vi "Sub_post_processing.vi"(0 "Experiment":T1, 1 "file name":i32, 2 "Save Acceleration Data":bool) -> (7 "Frequency":waveform(dbl)[](array[waveform]), 8 "Position":waveform(dbl)[](array[waveform]), 9 "average cycle time (ms)":dbl=4.283940110367686 format="%0.2f")   [LabVIEW 2021]
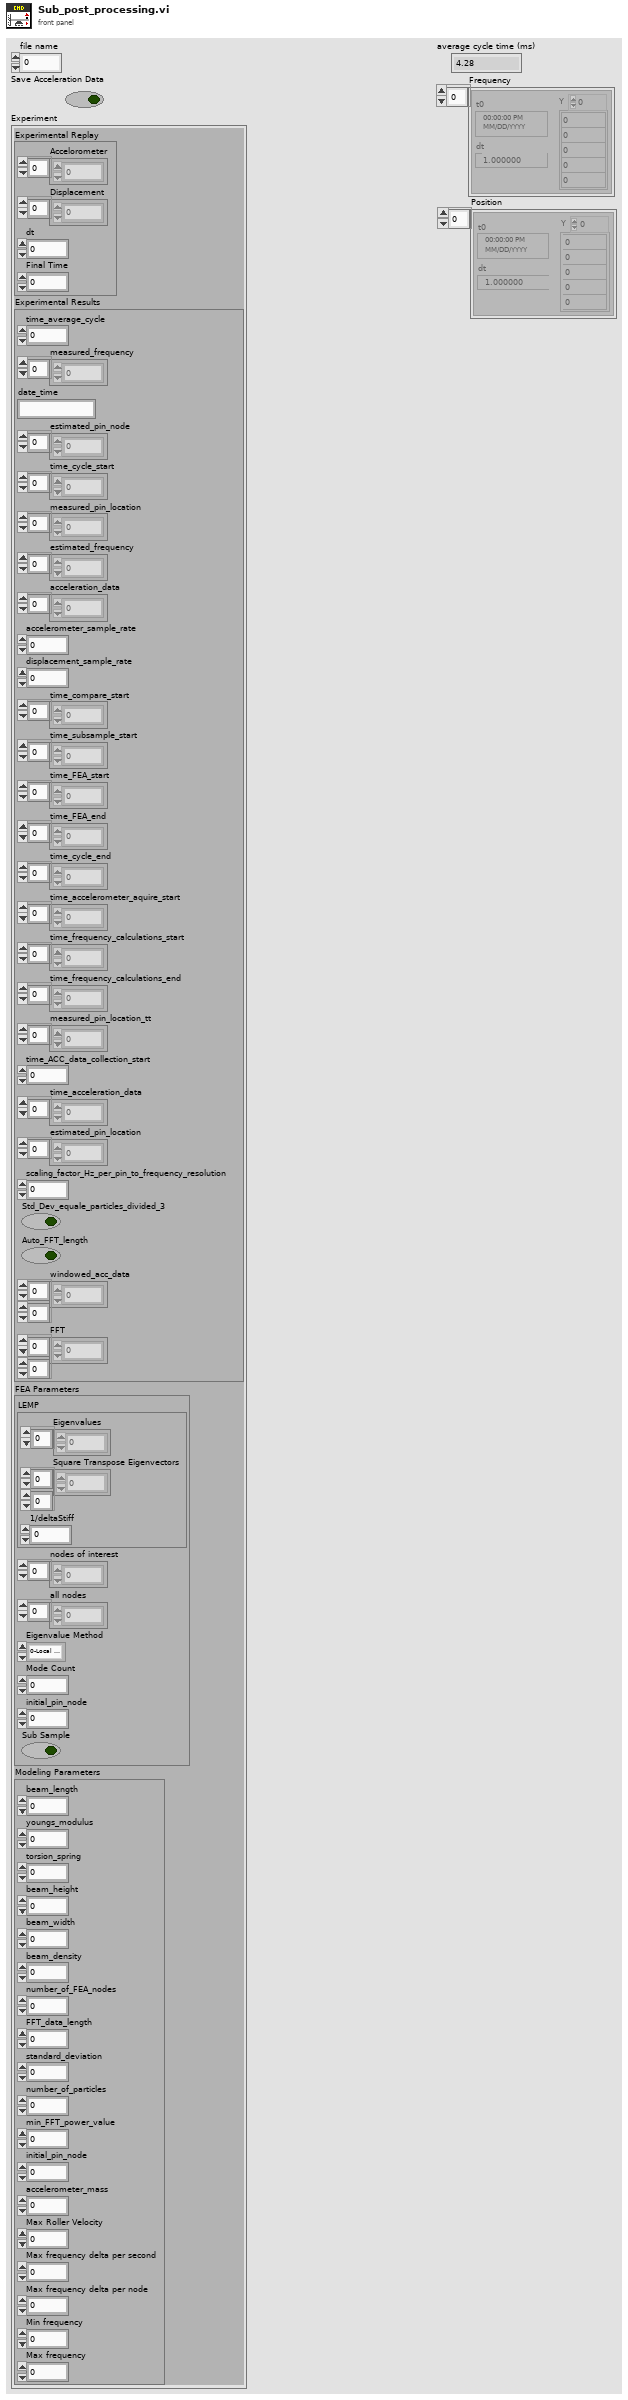
[diagram p1: front panel]
types:
  T1 = cluster{"Experimental Replay":cluster{"Accelorometer":dbl[], "Displacement":dbl[], "dt":dbl, "Final Time":dbl}, "Experimental Results":cluster{"time_average_cycle":dbl, "measured_frequency":dbl[], "date_time":string, "estimated_pin_node":i32[], "time_cycle_start":dbl[], "measured_pin_location":dbl[], "estimated_frequency":dbl[], "acceleration_data":dbl[], "accelerometer_sample_rate":dbl, "displacement_sample_rate":dbl, "time_compare_start":dbl[], "time_subsample_start":dbl[], "time_FEA_start":dbl[], "time_FEA_end":dbl[], "time_cycle_end":dbl[], "time_accelerometer_aquire_start":dbl[], "time_frequency_calculations_start":dbl[], "time_frequency_calculations_end":dbl[], "measured_pin_location_tt":dbl[], "time_ACC_data_collection_start":dbl, "time_acceleration_data":dbl[], "estimated_pin_location":dbl[], "scaling_factor_Hz_per_pin_to_frequency_resolution":dbl, "Std_Dev_equale_particles_divided_3":bool, "Auto_FFT_length":bool, "windowed_acc_data":dbl[][], "FFT":dbl[][]}, "FEA Parameters":cluster{"LEMP":cluster{"Eigenvalues":dbl[], "Square Transpose Eigenvectors":dbl[][], "1/deltaStiff":dbl}, "nodes of interest":i32[], "all nodes":i32[], "Eigenvalue Method":enum16{"0-Local Eigen Modification Procedure", "1-LabVIEW generalized eigenvalues", "2-LabVIEW M^-1K eigenvalues", "3-LabVIEW Cholesky Factorization", "4-Cholesky Factorization CPU SGL", "5-Cholesky Factorization CPU FXP", "6-Cholesky Factorization FPGA SGL", "7-Cholesky Factorization FPGA SGL SCL"}, "Mode Count":i32, "initial_pin_node":i32, "Sub Sample":bool}, "Modeling Parameters":cluster{"beam_length":dbl, "youngs_modulus":dbl, "torsion_spring":dbl, "beam_height":dbl, "beam_width":dbl, "beam_density":dbl, "number_of_FEA_nodes":i32, "FFT_data_length":i32, "standard_deviation":dbl, "number_of_particles":i32, "min_FFT_power_value":dbl, "initial_pin_node":i32, "accelerometer_mass":dbl, "Max Roller Velocity":dbl, "Max frequency delta per second":dbl, "Max frequency delta per node":dbl, "Min frequency":dbl, "Max frequency":dbl}}
  T2 = cluster{"beam_length":dbl, "youngs_modulus":dbl, "torsion_spring":dbl, "beam_height":dbl, "beam_width":dbl, "beam_density":dbl, "number_of_FEA_nodes":i32, "FFT_data_length":i32, "standard_deviation":dbl, "number_of_particles":i32, "min_FFT_power_value":dbl, "initial_pin_node":i32, "accelerometer_mass":dbl, "Max Roller Velocity":dbl, "Max frequency delta per second":dbl, "Max frequency delta per node":dbl, "Min frequency":dbl, "Max frequency":dbl}
  T3 = cluster{"time_average_cycle":dbl, "measured_frequency":dbl[], "date_time":string, "estimated_pin_node":i32[], "time_cycle_start":dbl[], "measured_pin_location":dbl[], "estimated_frequency":dbl[], "acceleration_data":dbl[], "accelerometer_sample_rate":dbl, "displacement_sample_rate":dbl, "time_compare_start":dbl[], "time_subsample_start":dbl[], "time_FEA_start":dbl[], "time_FEA_end":dbl[], "time_cycle_end":dbl[], "time_accelerometer_aquire_start":dbl[], "time_frequency_calculations_start":dbl[], "time_frequency_calculations_end":dbl[], "measured_pin_location_tt":dbl[], "time_ACC_data_collection_start":dbl, "time_acceleration_data":dbl[], "estimated_pin_location":dbl[], "scaling_factor_Hz_per_pin_to_frequency_resolution":dbl, "Std_Dev_equale_particles_divided_3":bool, "Auto_FFT_length":bool, "windowed_acc_data":dbl[][], "FFT":dbl[][]}
  T4 = cluster{"time_average_cycle":dbl, "measured_frequency":dbl[], "date_time":string, "estimated_pin_node":i32[], "time_cycle_start":dbl[], "measured_pin_location":dbl[], "estimated_frequency":dbl[], "acceleration_data":dbl[], "accelerometer_sample_rate":dbl, "displacement_sample_rate":dbl, "time_compare_start":dbl[], "time_subsample_start":dbl[], "time_FEA_start":dbl[], "time_FEA_end":dbl[], "time_cycle_end":dbl[], "time_accelerometer_aquire_start":dbl[], "time_frequency_calculations_start":dbl[], "time_frequency_calculations_end":dbl[], "measured_pin_location_tt":dbl[], "time_ACC_data_collection_start":dbl, "time_acceleration_data":dbl[], "estimated_pin_location":dbl[], "scaling_factor_Hz_per_pin_to_frequency_resolution":dbl, "Std_Dev_equale_particles_divided_3":bool, "Auto_FFT_length":bool, "windowed_acc_data":dbl[][], "FFT":dbl[][], "beam_length":dbl, "youngs_modulus":dbl, "torsion_spring":dbl, "beam_height":dbl, "beam_width":dbl, "beam_density":dbl, "number_of_FEA_nodes":i32, "FFT_data_length":i32, "standard_deviation":dbl, "number_of_particles":i32, "min_FFT_power_value":dbl, "initial_pin_node":i32, "accelerometer_mass":dbl}
  T5 = cluster{"measured_pin_location_tt":dbl[], "measured_pin_location":dbl[]}
  T6 = cluster{"time_acceleration_data":dbl[], "acceleration_data":dbl[]}
  T7 = cluster{"time_cycle_end":dbl[], "estimated_pin_location":dbl[]}
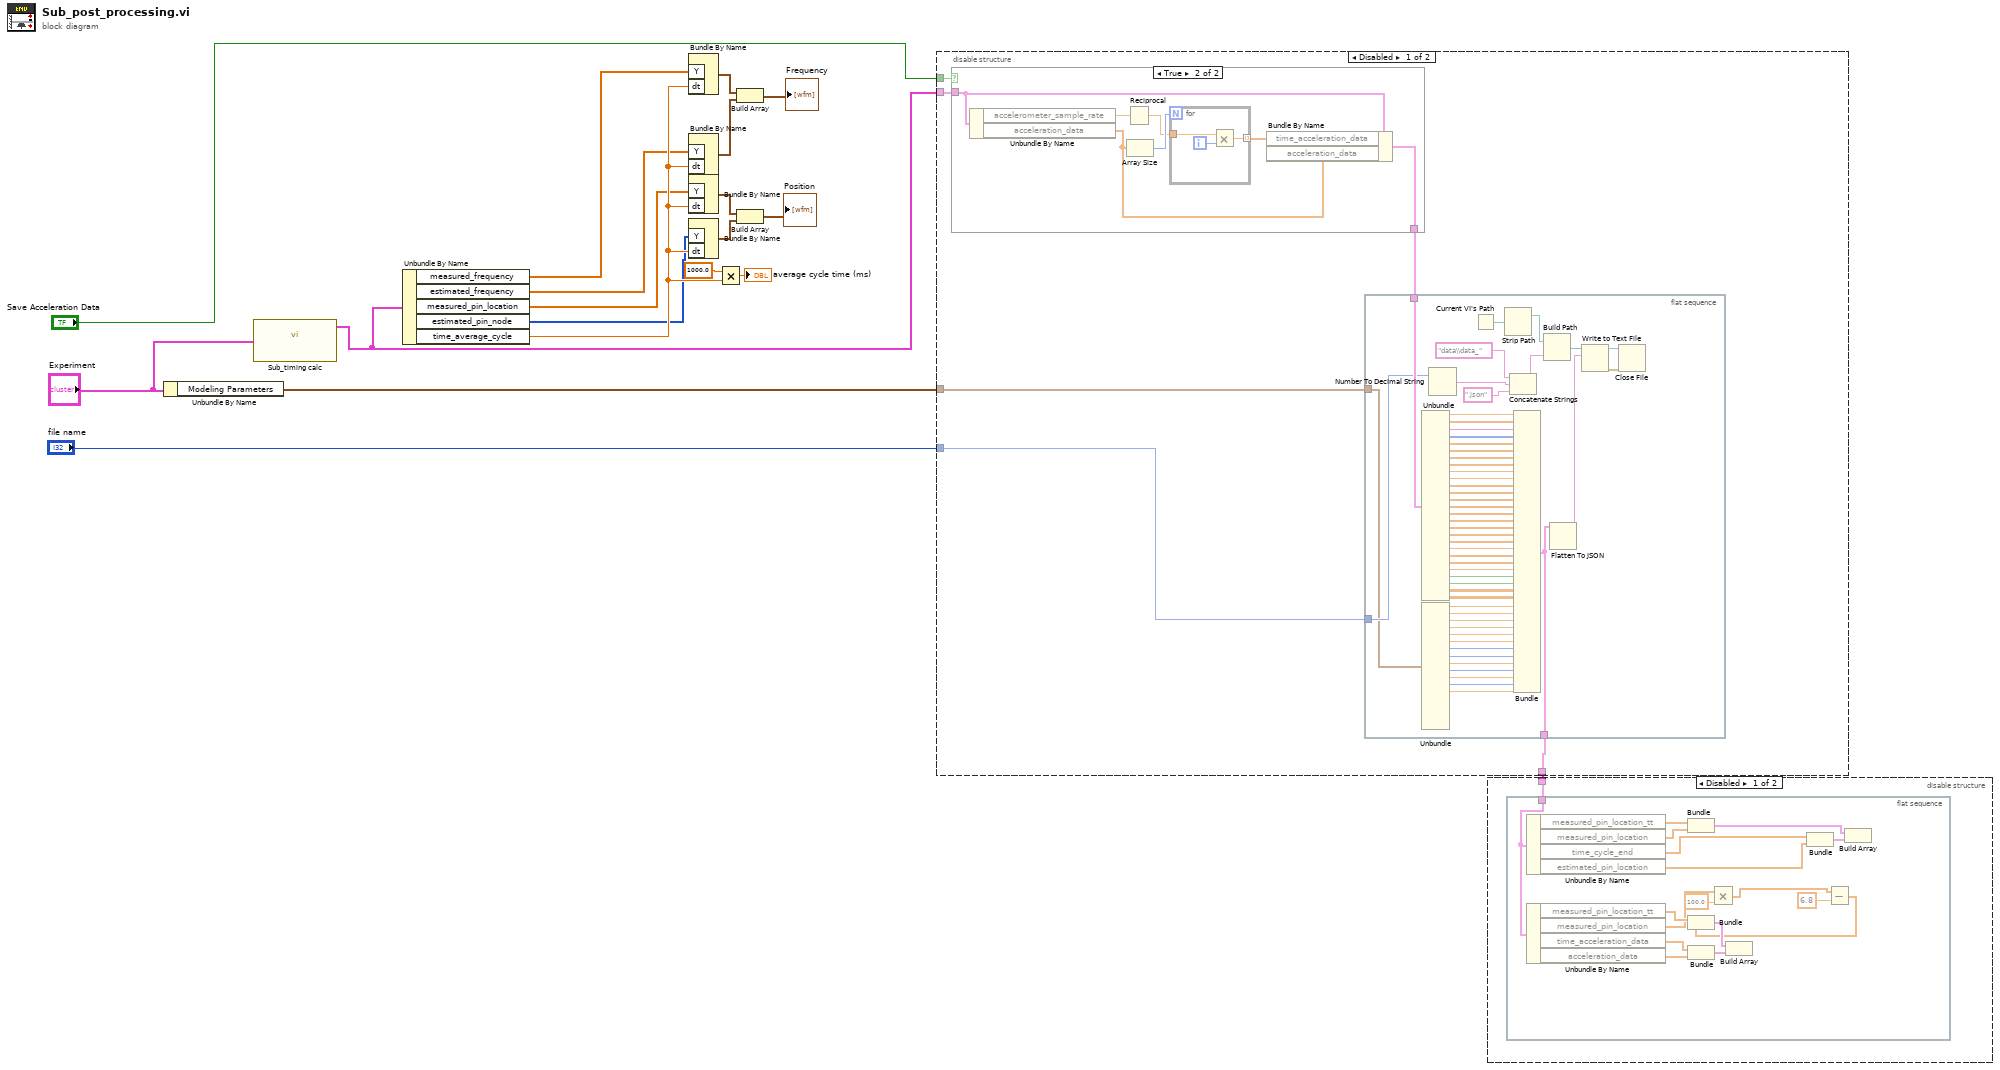
[diagram p0: block diagram]
diagram:
  n1 = Unbundle By Name("Experiment") -> ("Modeling Parameters"=w2:T2)
  n2 = call "Sub_timing calc.vi"("Experiment In"="Experiment") -> ("Experimental Results OUT"=w7:T3)  [unwired: 1 out]
  n3 = Unbundle By Name(w7) -> ("measured_frequency"=w6:dbl[], "estimated_frequency"=w5:dbl[], "measured_pin_location"=w4:dbl[], "estimated_pin_node"=w3:i32[], "time_average_cycle"=w8:dbl)
  n4 = Bundle By Name("Y"=w6, "dt"=w8) -> (w14:waveform(dbl))  [unwired: 1 in]
  n5 = Bundle By Name("Y"=w5, "dt"=w8) -> (w13:waveform(dbl))  [unwired: 1 in]
  n6 = Bundle By Name("Y"=w4, "dt"=w8) -> (w11:waveform(dbl))  [unwired: 1 in]
  n7 = Bundle By Name("Y"=w3, "dt"=w8) -> (w10:waveform(i32))  [unwired: 1 in]
  n8 = Multiply(x=1000.0, y=w8) -> (x*y=→"average cycle time (ms)":dbl)
  n9 = Build Array(w14, w13) -> (→"Frequency":waveform(dbl)[])
  n10 = Build Array(w11, w10) -> (→"Position":waveform(dbl)[])
  n11 = disable-structure shown="Disabled" {
    disable-tunnel: "file name" -> [w25 _]
    disable-tunnel: [w24 _] -> w16
    disable-tunnel: "Save Acceleration Data" -> [w23 _]
    disable-tunnel: w7 -> [w21 _]
    disable-tunnel: w2 -> [w20 _]
    frame Disabled {
      n12 = case shown="True" w23 {
        tunnel: [w26 w33] -> w22
        tunnel: w21 -> [w26 w32]
        frame False {
        }
        frame True {
          n13 = Unbundle By Name(w32) -> ("accelerometer_sample_rate"=w28:dbl, "acceleration_data"=w27:dbl[])
          n14 = Reciprocal(x=w28) -> (1/x=w29:dbl)
          n15 = Array Size(array=w27) -> (size(s)=w30:i32)
          n16 = for {
            N: w30 -> [_]
            tunnel: w29 -> [w35]
            tunnel: [w34] -> w31 mode=indexing
            i -> [w36]
            n17 = Multiply(x=w35, y=w36) -> (x*y=w34:dbl)
          }
          n18 = Bundle By Name(cluster=w32, "time_acceleration_data"=w31, "acceleration_data"=w27) -> (w33:T3)
        }
      }
      n19 = flat-sequence {
        tunnel: w22 -> [w63]
        tunnel: w25 -> [w58]
        tunnel: [w56] -> w24
        tunnel: w20 -> [w37]
        frame #0 {
          n20 = Unbundle(w63) -> ("time_average_cycle"=w67:dbl, "measured_frequency"=w68:dbl[], "date_time"=w69:string, "estimated_pin_node"=w70:i32[], "time_cycle_start"=w71:dbl[], "measured_pin_location"=w72:dbl[], "estimated_frequency"=w73:dbl[], "acceleration_data"=w74:dbl[], "accelerometer_sample_rate"=w75:dbl, "displacement_sample_rate"=w76:dbl, "time_compare_start"=w77:dbl[], "time_subsample_start"=w78:dbl[], "time_FEA_start"=w79:dbl[], "time_FEA_end"=w80:dbl[], "time_cycle_end"=w81:dbl[], "time_accelerometer_aquire_start"=w82:dbl[], "time_frequency_calculations_start"=w83:dbl[], "time_frequency_calculations_end"=w84:dbl[], "measured_pin_location_tt"=w66:dbl[], "time_ACC_data_collection_start"=w65:dbl, "time_acceleration_data"=w64:dbl[], "estimated_pin_location"=w57:dbl[], "scaling_factor_Hz_per_pin_to_frequency_resolution"=w55:dbl, "Std_Dev_equale_particles_divided_3"=w54:bool, "Auto_FFT_length"=w53:bool, "windowed_acc_data"=w52:dbl[][], "FFT"=w51:dbl[][])
          n21 = Unbundle(w37) -> ("beam_length"=w50:dbl, "youngs_modulus"=w49:dbl, "torsion_spring"=w48:dbl, "beam_height"=w47:dbl, "beam_width"=w46:dbl, "beam_density"=w45:dbl, "number_of_FEA_nodes"=w44:i32, "FFT_data_length"=w43:i32, "standard_deviation"=w42:dbl, "number_of_particles"=w41:i32, "min_FFT_power_value"=w40:dbl, "initial_pin_node"=w39:i32, "accelerometer_mass"=w38:dbl)  [unwired: 5 out]
          n22 = Number To Decimal String(number=w58) -> (decimal integer string=w59:string)  [unwired: 1 in]
          n23 = Current VI's Path() -> (path=w87:path)
          n24 = Strip Path(path=w87) -> (stripped path=w86:path)  [unwired: 1 out]
          n25 = Concatenate Strings("data\\data_" ("name or relative path"), w59, ".json" ("name or relative path")) -> (w60:string)
          n26 = Bundle("time_average_cycle"=w67, "measured_frequency"=w68, "date_time"=w69, "estimated_pin_node"=w70, "time_cycle_start"=w71, "measured_pin_location"=w72, "estimated_frequency"=w73, "acceleration_data"=w74, "accelerometer_sample_rate"=w75, "displacement_sample_rate"=w76, "time_compare_start"=w77, "time_subsample_start"=w78, "time_FEA_start"=w79, "time_FEA_end"=w80, "time_cycle_end"=w81, "time_accelerometer_aquire_start"=w82, "time_frequency_calculations_start"=w83, "time_frequency_calculations_end"=w84, "measured_pin_location_tt"=w66, "time_ACC_data_collection_start"=w65, "time_acceleration_data"=w64, "estimated_pin_location"=w57, "scaling_factor_Hz_per_pin_to_frequency_resolution"=w55, "Std_Dev_equale_particles_divided_3"=w54, "Auto_FFT_length"=w53, "windowed_acc_data"=w52, "FFT"=w51, "beam_length"=w50, "youngs_modulus"=w49, "torsion_spring"=w48, "beam_height"=w47, "beam_width"=w46, "beam_density"=w45, "number_of_FEA_nodes"=w44, "FFT_data_length"=w43, "standard_deviation"=w42, "number_of_particles"=w41, "min_FFT_power_value"=w40, "initial_pin_node"=w39, "accelerometer_mass"=w38) -> (w56:T4)  [unwired: 1 in]
          n27 = Build Path(base path=w86, name or relative path=w60) -> (appended path=w85:path)
          n28 = Flatten To JSON(anything=w56) -> (JSON string=w88:string)  [unwired: 2 in, 1 out]
          n29 = Write to Text File(file (use dialog)=w85, text=w88) -> (refnum out=w90:refnum<file>, error out=w89:errorcluster)  [unwired: 2 in, 1 out]
          n30 = Close File(refnum=w90, error in=w89) -> ()  [unwired: 2 out]
        }
      }
    }
    frame Enabled {
    }
  }
  n31 = disable-structure shown="Disabled" {
    disable-tunnel: w16 -> [w91 _]
    frame Disabled {
      n32 = flat-sequence {
        tunnel: w91 -> [w96]
        frame #0 {
          n33 = Unbundle By Name(w96) -> ("measured_pin_location_tt"=w107:dbl[], "measured_pin_location"=w95:dbl[], "time_cycle_end"=w106:dbl[], "estimated_pin_location"=w94:dbl[])
          n34 = Unbundle By Name(w96) -> ("measured_pin_location_tt"=w105:dbl[], "measured_pin_location"=w101:dbl[], "time_acceleration_data"=w92:dbl[], "acceleration_data"=w103:dbl[])
          n35 = Bundle("measured_pin_location_tt"=w107, "measured_pin_location"=w95) -> (w108:T5)  [unwired: 1 in]
          n36 = Bundle("time_acceleration_data"=w92, "acceleration_data"=w103) -> (w102:T6)  [unwired: 1 in]
          n37 = Multiply(x=w101, y=100.0 ("x")) -> (x*y=w98:dbl[])
          n38 = Bundle("time_cycle_end"=w106, "estimated_pin_location"=w94) -> (w93:T7)  [unwired: 1 in]
          n39 = Subtract(x=w98, y=6.8) -> (x-y=w97:dbl[])
          n40 = Bundle("measured_pin_location_tt"=w105, w97) -> (w104:cluster{"measured_pin_location_tt":dbl[], dbl[]})  [unwired: 1 in]
          n41 = Build Array(w104, w102) -> ()  [unwired: 1 out]
          n42 = Build Array(w108, w93) -> ()  [unwired: 1 out]
        }
      }
    }
    frame Enabled {
    }
  }
